vi "PowerConvertor.vi"(10 "Power In":u16, 11 "Action":enum16{"Get power (%)", "Get Power (Unite)"}(ring)) -> (3 "Power Out":u16)   [LabVIEW 2017]
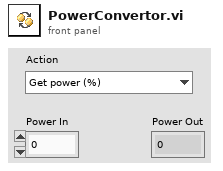
[diagram p1: front panel]
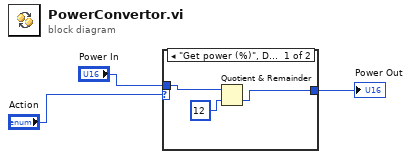
[diagram p0: block diagram]
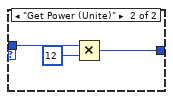
[diagram p2: hidden frame]
diagram:
  n1 = case shown="\"Get power (%)\", Default" "Action" {
    tunnel: "Power In" -> [w6 w9]
    tunnel: [w4 w7] -> w2
    frame "Get power (%)", Default {
      n2 = Quotient & Remainder(x=w6, y=u8 12) -> (floor(x/y)=w4:u16)  [unwired: 1 out]
    }
    frame "Get Power (Unite)" {
      n3 = Multiply(x=w9, y=u8 12) -> (x*y=w7:u16)
    }
  }
  "Power Out" <- w2
